vi "get_shutter.vi"(8 "error in (no error)":errorcluster, 11 "LightSourceMH110125Tsunami in":refnum<class "LightSourceMH110125Tsunami.lvclass">) -> (0 "error out":errorcluster, 2 "shutter open out?":bool, 3 "LightSourceMH110125Tsunami out":refnum<class "LightSourceMH110125Tsunami.lvclass">)   [LabVIEW 2010, in "LightSourceMH110125Tsunami.lvclass"]
uses:
  LightSourceMH110125Tsunami.lvclass
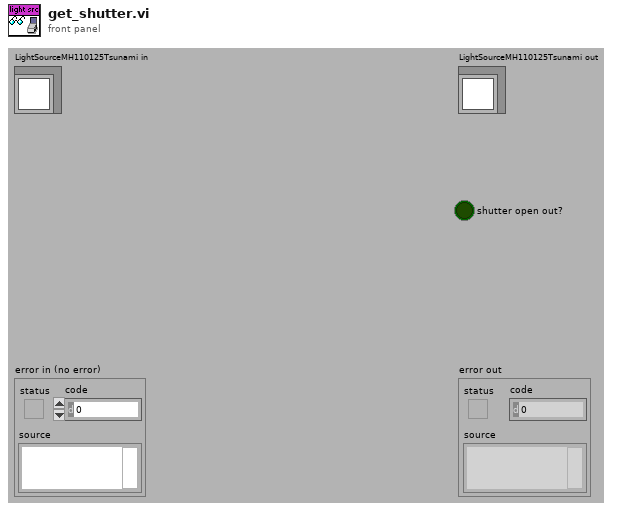
[diagram p1: front panel]
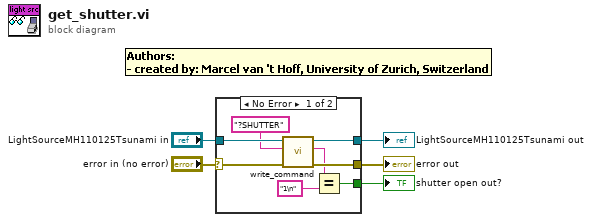
[diagram p0: block diagram]
diagram:
  n1 = case shown="No Error" "error in (no error)" {
    selector: "error in (no error)" -> [w11 w14]
    tunnel: [w10 w14] -> w4
    tunnel: [w12 w15] -> w2
    tunnel: "LightSourceMH110125Tsunami in" -> [w13 w15]
    tunnel: [w6 _] -> w1
    frame No Error {
      n2 = call-dynamic "write_command.vi"("error in (no error)"=w11, "string to write"="?SHUTTER", "LightSourceMH110125Tsunami in"=w13) -> ("error out"=w10:errorcluster, "read string"=w7:string, "LightSourceMH110125Tsunami out"=w12:refnum<class "LightSourceMH110125Tsunami.lvclass">)  [unwired: 6 in]
      n3 = Equal?(x=w7, y="1\n") -> (x = y?=w6:bool)
    }
    frame Error {
    }
  }
  "error out" <- w4
  "LightSourceMH110125Tsunami out" <- w2
  "shutter open out?" <- w1
